vi "PNS VisBx Simulation mit Enum.vi"   [LabVIEW 2015, in "Anlagenuebersicht.lvlib"]
uses:
  Anlagenuebersicht.lvlib
  PNS Uebersicht.ctl
types:
  T1 = typedef "Anlagenuebersicht.lvlib/PNS Uebersicht.ctl" = cluster{"VFS 1 Y1":bool, "VFS 1 Y2":bool, "VFS 1 Y3":bool, "VFS 1 Y4":bool, "VFS 1 Y Reserve1":bool, "VFS 1 Y Reserve2":bool, "VFS 2 Y1":bool, "VFS 2 Y2":bool, "VFS 2 Y3":bool, "VFS 2 Y4":bool, "VFS 2 Y Reserve1":bool, "VFS 2 Y Reserve2":bool, "VFS 3 Y1":bool, "VFS 3 Y2":bool, "VFS 3 Y3":bool, "VFS 3 Y4":bool, "VFS 3 Y Reserve1":bool, "VFS 3 Y Reserve2":bool, "VFS 4 Y1":bool, "VFS 4 Y2":bool, "VFS 4 Y3":bool, "VFS 4 Y4":bool, "VFS 4 Y Reserve1":bool, "VFS 4 Y Reserve2":bool, "Zustand":enum16{"Stby/Pause/Eco", "Messen", "Spülen Filter", "Spülen Leitung", "Umgebungsluft", "0-Gas / Hintergrund", "Cal-Gas"}}
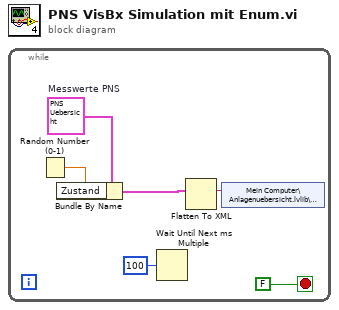
[diagram p0: block diagram]
diagram:
  n1 = while {
    stop <- FALSE stop-if-true
    w2 = T1 {"VFS 1 Y1"=FALSE, "VFS 1 Y2"=FALSE, "VFS 1 Y3"=FALSE, "VFS 1 Y4"=FALSE, "VFS 1 Y Reserve1"=FALSE, "VFS 1 Y Reserve2"=FALSE, "VFS 2 Y1"=FALSE, "VFS 2 Y2"=FALSE, "VFS 2 Y3"=FALSE, "VFS 2 Y4"=FALSE, "VFS 2 Y Reserve1"=FALSE, "VFS 2 Y Reserve2"=FALSE, "VFS 3 Y1"=FALSE, "VFS 3 Y2"=FALSE, "VFS 3 Y3"=FALSE, "VFS 3 Y4"=FALSE, "VFS 3 Y Reserve1"=FALSE, "VFS 3 Y Reserve2"=FALSE, "VFS 4 Y1"=FALSE, "VFS 4 Y2"=FALSE, "VFS 4 Y3"=FALSE, "VFS 4 Y4"=FALSE, "VFS 4 Y Reserve1"=FALSE, "VFS 4 Y Reserve2"=FALSE, "Zustand"=enum."Stby/Pause/Eco"}  # Messwerte PNS
    n2 = Random Number (0-1)() -> (number: 0 to 1=w3:dbl)
    n3 = Bundle By Name(cluster=w2, "Zustand"=w3) -> (w4:T1)
    n4 = Wait Until Next ms Multiple(millisecond multiple=u32 100 ("Vielfache von ms")) -> ()  [unwired: 1 out]
    n5 = Flatten To XML(anything=w4) -> (xml string=w1:string)
    n6 = shared-variable "Mein Computer\\Anlagenuebersicht.lvlib\\VisDat PNS"(w1) -> ()  [unwired: 1 in, 1 out]
  }
